vi "Corr Find Relative Pth.vi"(1 "INFO path":path, 2 "CSV path":path) -> (0 "CSV relative path":string)   [LabVIEW 2013]
doc: "Converts absolute CSV path to relative from the INFO path."
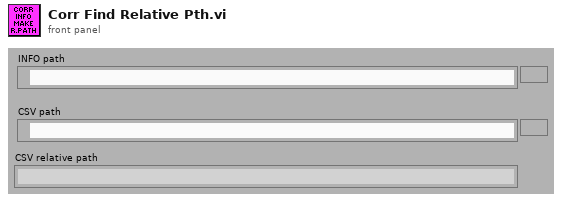
[diagram p1: front panel]
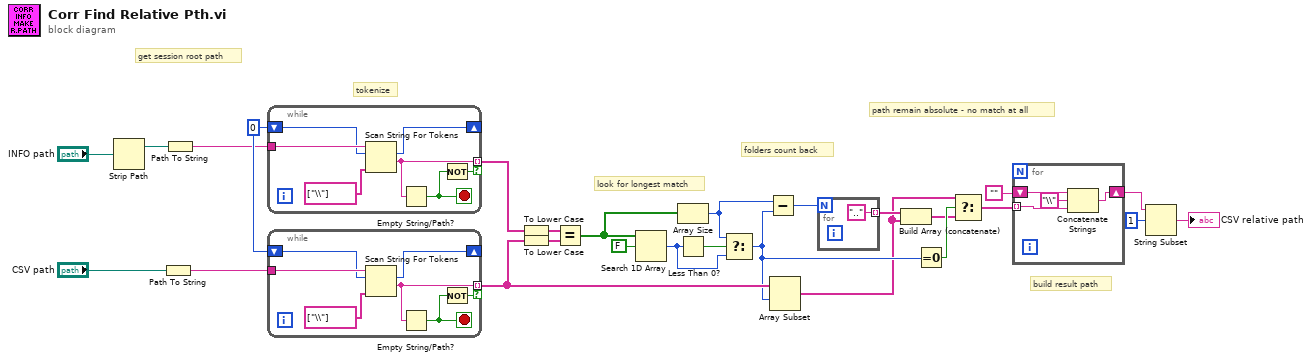
[diagram p0: block diagram]
diagram:
  w24 = 0 ("offset past token")
  # "build result path"
  # "path remain absolute - no match at all"
  # "look for longest match"
  # "tokenize"
  # "folders count back"
  # "get session root path"
  n1 = Strip Path(path="INFO path") -> (stripped path=w23:path)  [unwired: 1 out]
  n2 = Path To String(path="CSV path") -> (string=w3:string)
  n3 = Path To String(path=w23) -> (string=w4:string)
  n4 = while {
    tunnel: w4 -> [w33]
    shift-right: [w30] -> _
    shift-left: w24 -> [w31]
    tunnel: [w29] -> w22 mode=indexing if=w28
    stop <- w27 stop-if-true
    n5 = Scan String For Tokens(6:string[] ["\\"] ("delimiters (\\s,\\t,\\r,\\n)"), 8:w31, 9:w33) -> (1:w29:string, 2:w30:i32)  [unwired: 3 in, 2 out]
    n6 = Empty String/Path?(string/path=w29) -> (empty?=w27:bool)
    n7 = Not(x=w27) -> (.not. x?=w28:bool)
  }
  n8 = while {
    tunnel: w3 -> [w40]
    shift-right: [w37] -> _
    shift-left: w24 -> [w38]
    tunnel: [w36] -> w17 mode=indexing if=w35
    stop <- w34 stop-if-true
    n9 = Scan String For Tokens(6:string[] ["\\"] ("delimiters (\\s,\\t,\\r,\\n)"), 8:w38, 9:w40) -> (1:w36:string, 2:w37:i32)  [unwired: 3 in, 2 out]
    n10 = Empty String/Path?(string/path=w36) -> (empty?=w34:bool)
    n11 = Not(x=w34) -> (.not. x?=w35:bool)
  }
  n12 = To Lower Case(string=w22) -> (all lower case string=w2:string[])
  n13 = To Lower Case(string=w17) -> (all lower case string=w1:string[])
  n14 = Equal?(x=w2, y=w1) -> (x = y?=w19:bool[])
  n15 = Search 1D Array(1D array=w19, element=FALSE) -> (index of element=w18:i32)  [unwired: 1 in]
  n16 = Array Size(array=w19) -> (size(s)=w16:i32)
  n17 = Less Than 0?(x=w18) -> (x < 0?=w20:bool)
  n18 = Select(t=w16, s=w20, f=w18) -> (s? t:f=w13:i32)
  n19 = Subtract(x=w16, y=w13) -> (x-y=w15:i32)
  n20 = Array Subset(array=w17, index=w13) -> (w10:string[])  [unwired: 1 in]
  n21 = for {
    N: w15 -> [_]
    tunnel: [".."] -> w14 mode=indexing
  }
  n22 = Build Array (concatenate)(w14, w10) -> (w11:string[])
  n23 = Equal To 0?(x=w13) -> (x = 0?=w12:bool)
  n24 = Select(t=w10, s=w12, f=w11) -> (s? t:f=w9:string[])
  n25 = for {
    tunnel: w9 -> [w44] mode=indexing
    shift-right: [w42] -> w7
    shift-left: "" -> [w45]
    n26 = Concatenate Strings(w45, "\\" ("string"), w44) -> (w42:string)
  }
  n27 = String Subset(string=w7, offset (0)=1) -> (substring=→"CSV relative path":string)  [unwired: 1 in]
